vi "Read Index Mode.vi"(9 "LoopTunnel in":refnum<class "LoopTunnel.lvclass">) -> (3 "LoopTunnel out":refnum<class "LoopTunnel.lvclass">, 4 "Index Mode":u32)   [LabVIEW 2014, in "LoopTunnel.lvclass"]
uses:
  LoopTunnel.lvclass
  LoopTunnel.lvclass/LoopTunnel.ctl
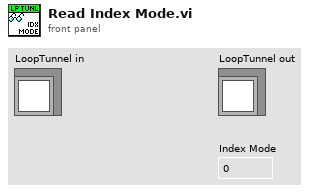
[diagram p1: front panel]
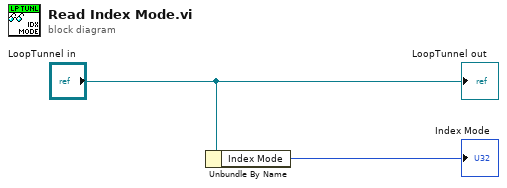
[diagram p0: block diagram]
diagram:
  n1 = Unbundle By Name("LoopTunnel in") -> ("Index Mode"=→"Index Mode":u32)
  "LoopTunnel out" <- "LoopTunnel in"
